vi "Write Camera Configuration.vi"(8 "error in (no error)":errorcluster, 10 "CCD Config":T1={"Image Path"="C:\\Users\\Cliente\\Desktop\\SPARC4_AC\\Imagens\\", "Image Name"="Image", "Exposure Time"=0.0, "Pre-amp gain"=0, "Readout Rate"=0, "EM Mode"=0, "EM Gain"=2, "Binning"=1, "Initial Line"=1, "Initial Cloumn"=1, "Final Line"=1024, "Final Column"=1024, "Kinetic Series Length"=0, "Shutter Mode"=2, "Cooler ON/OFF"=0, "Temperature"=20} {"Temperature" min=0 max=0; "Cooler ON/OFF" items=["Cooler OFF", "Cooler ON"]; "Shutter Mode" items=["Fully Auto", "OPEN", "CLOSED"]; "EM Mode" items=["Electron Multiplying", "Conventional"]; "Readout Rate" items=["1 MHz", "10 MHz", "20 MHz", "30 MHz"]; "Pre-amp gain" items=["Gain 1", "Gain 2"]}, 11 "CCDCamera in":refnum<class "Simulated_CCD_Camera.lvclass">) -> (0 "error out":errorcluster, 3 "CCDCamera out":refnum<class "Simulated_CCD_Camera.lvclass">)   [LabVIEW 2018, in "Simulated_CCD_Camera.lvclass"]
uses:
  Simulated_CCD_Camera.lvclass
  Simulated_CCD_Camera.lvclass/Simulated_CCD_Camera.ctl
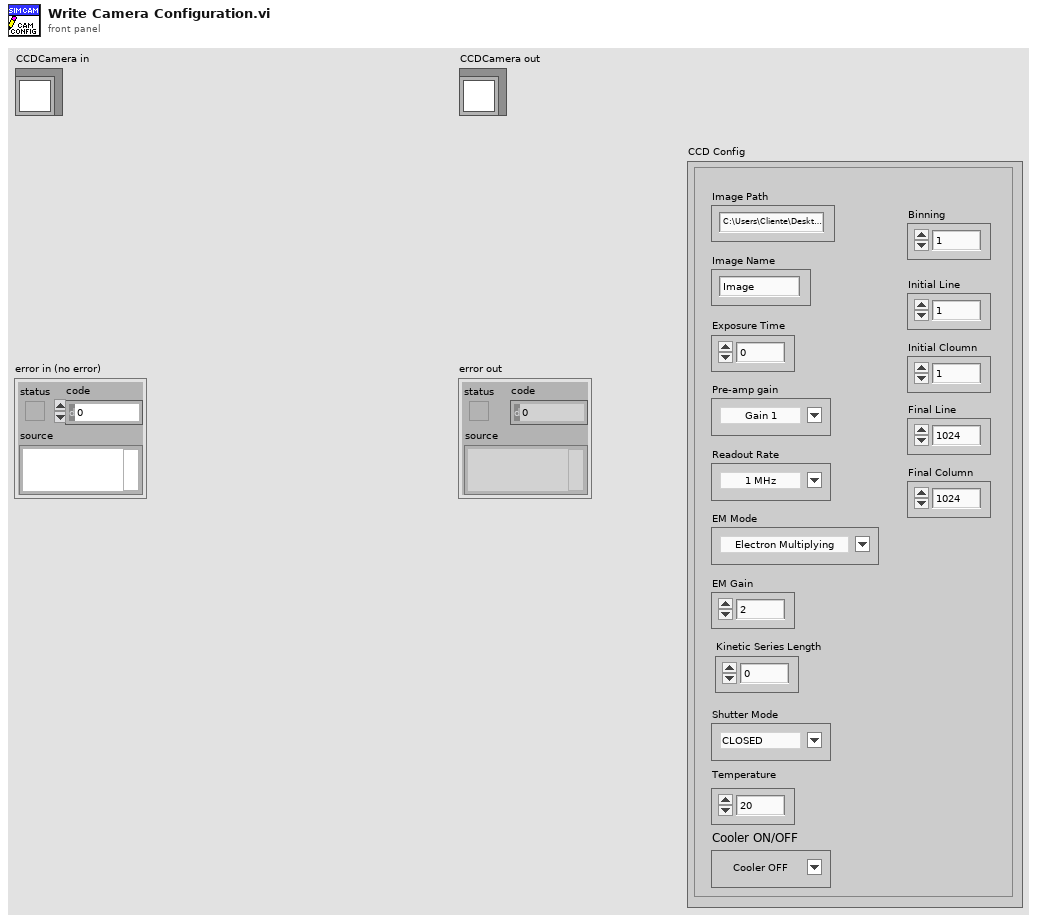
[diagram p1: front panel]
types:
  T1 = cluster{"Image Path":string, "Image Name":string, "Exposure Time":sgl, "Pre-amp gain":u8, "Readout Rate":u8, "EM Mode":u8, "EM Gain":u16, "Binning":u16, "Initial Line":u16, "Initial Cloumn":u16, "Final Line":u16, "Final Column":u16, "Kinetic Series Length":u32, "Shutter Mode":u8, "Cooler ON/OFF":u16, "Temperature":i8}
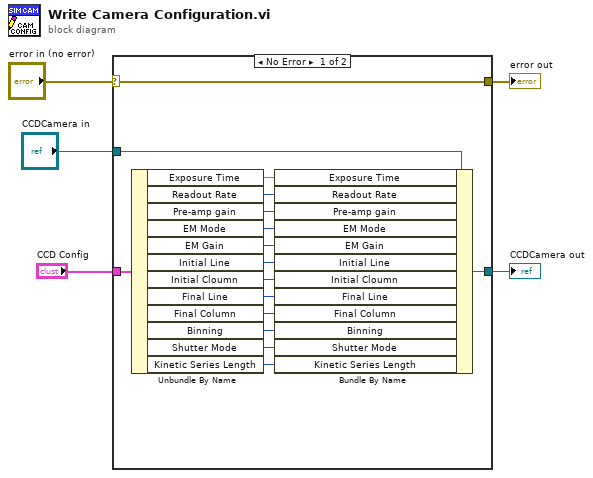
[diagram p0: block diagram]
diagram:
  n1 = case shown="No Error" "error in (no error)" {
    selector: "error in (no error)" -> [w10 w22]
    tunnel: [w10 w22] -> w4
    tunnel: [w9 w23] -> w2
    tunnel: "CCDCamera in" -> [w21 w23]
    tunnel: "CCD Config" -> [w20 _]
    frame No Error {
      n2 = Unbundle By Name(w20) -> ("Exposure Time"=w19:sgl, "Readout Rate"=w18:u8, "Pre-amp gain"=w17:u8, "EM Mode"=w16:u8, "EM Gain"=w15:u16, "Initial Line"=w14:u16, "Initial Cloumn"=w13:u16, "Final Line"=w12:u16, "Final Column"=w11:u16, "Binning"=w6:u16, "Shutter Mode"=w8:u8, "Kinetic Series Length"=w7:u32)
      n3 = Bundle By Name(cluster=w21, "Exposure Time"=w19, "Readout Rate"=w18, "Pre-amp gain"=w17, "EM Mode"=w16, "EM Gain"=w15, "Initial Line"=w14, "Initial Cloumn"=w13, "Final Line"=w12, "Final Column"=w11, "Binning"=w6, "Shutter Mode"=w8, "Kinetic Series Length"=w7) -> (w9:refnum<class "Simulated_CCD_Camera.lvclass">)
    }
    frame Error {
    }
  }
  "error out" <- w4
  "CCDCamera out" <- w2
